vi "PN_serie.vi"(11 "Frame Instruction 3":T1={"Code Rates"=4.0, "Length"=12.0, "Destination address"=8.0, "User"=2.0, "Source address "=12.0, " Frame number"=8.0, "Check Sum"=16.0}) -> (2 "同步大小":dbl, 3 "同步序列":bool[](array[boolean]))   [LabVIEW 2014]
uses:
  <vilib>/addons/Modulation/Digital/General/MT Generate Bits (Galois, PN Order).vi
  <vilib>/addons/Modulation/Digital/Support/Common/Validators/mod_Generate Bits Validate.vi
  <vilib>/addons/Modulation/Analog/support/mod_Set Error Source.vi
  <vilib>/addons/Modulation/Digital/General/subVIs/mod_Generate Bits PN Sequence.vi
  <vilib>/addons/Modulation/niDMT.lvlib
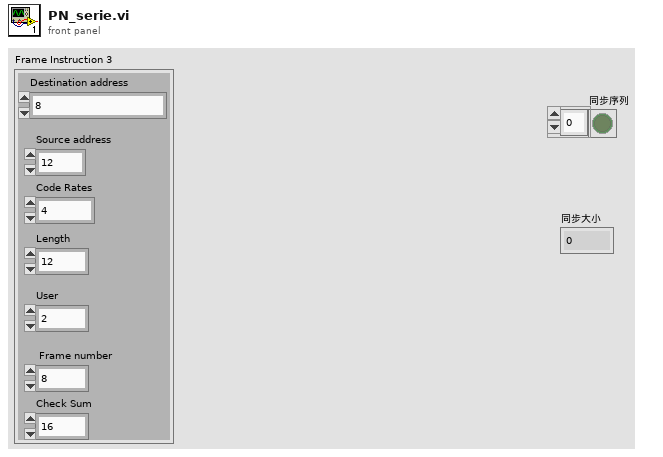
[diagram p1: front panel]
types:
  T1 = cluster{"Code Rates":dbl, "Length":dbl, "Destination address":dbl, "User":dbl, "Source address ":dbl, " Frame number":dbl, "Check Sum":dbl}
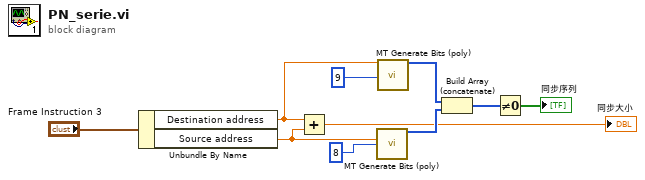
[diagram p0: block diagram]
diagram:
  n1 = Unbundle By Name("Frame Instruction 3") -> ("Destination address"=w5:dbl, "Source address"=w4:dbl)
  n2 = Add(x=w5, y=w4) -> (x+y=→"同步大小":dbl)
  n3 = call-poly <vilib>:"MT Generate Bits (poly).vi"("total bits (128)"=w4, "PN sequence order (9)"=8) -> ("output bit stream"=w7:i8[])  [unwired: 11 in, 2 out]
  n4 = call-poly <vilib>:"MT Generate Bits (poly).vi"("total bits (128)"=w5, "PN sequence order (9)"=9) -> ("output bit stream"=w8:i8[])  [unwired: 11 in, 2 out]
  n5 = Build Array (concatenate)(w8, w7) -> (w6:i8[])
  n6 = Not Equal To 0?(x=w6) -> (x != 0?=→"同步序列":bool[])
